vi "Launch Client.vi"(8 "error in":errorcluster, 10 "Client Name":string, 11 "Client Manager in":refnum<class "Client Manager.lvclass">) -> (0 "error out":errorcluster, 3 "Client Manager out":refnum<class "Client Manager.lvclass">)   [LabVIEW 2014, in "Client Manager.lvclass"]
uses:
  Client Manager.lvclass
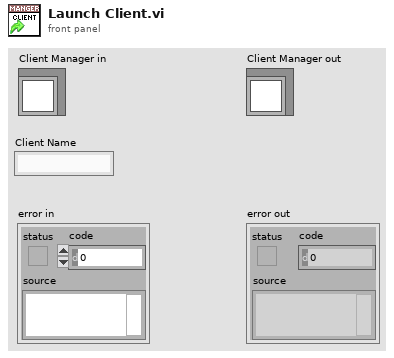
[diagram p1: front panel]
types:
  T1 = enum32{"Bad", "Idle", "Run top level", "Running"}
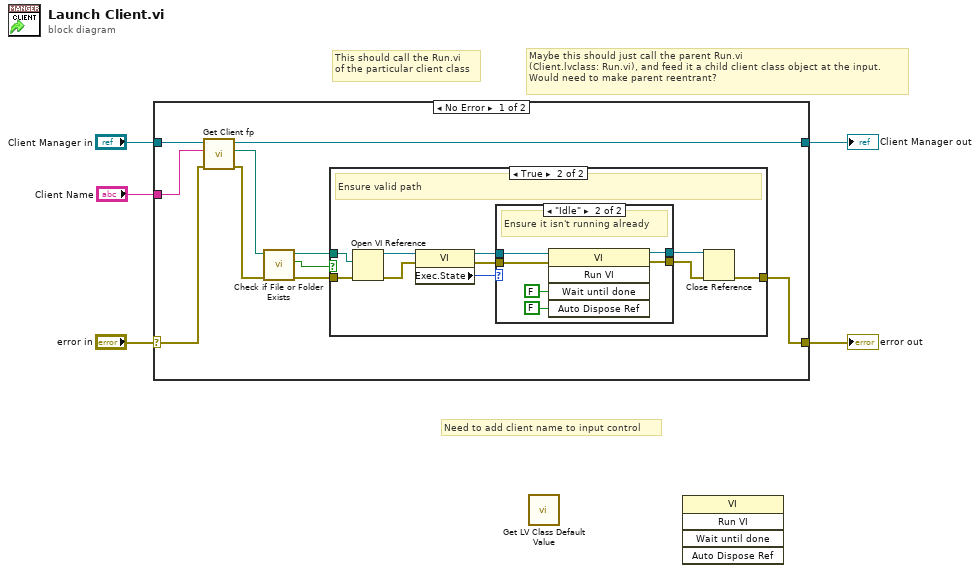
[diagram p0: block diagram]
diagram:
  # "Maybe this should just call the parent Run.vi \n(Client.lvclass: Run.vi), and feed it a child client class object at the input.\nWould need to make parent reentrant?"
  # "Need to add client name to input control"
  # "This should call the Run.vi\nof the particular client class"
  n1 = case shown="No Error" "error in" {
    selector: "error in" -> [w8 w36]
    tunnel: [w6 w36] -> w4
    tunnel: [w14 w35] -> w2
    tunnel: "Client Manager in" -> [w15 w35]
    tunnel: "Client Name" -> [w13 _]
    frame No Error {
      n2 = call "Get Client fp.vi"("error in"=w8, "Client Name"=w13, "Client Manager in"=w15) -> ("error out"=w7:errorcluster, "Client fp"=w12:path, "Client Manager out"=w14:refnum<class "Client Manager.lvclass">)  [unwired: 6 in]
      n3 = call <vilib>:"Check if File or Folder Exists.vi"("error in (no error)"=w7, "path"=w12) -> ("error out"=w9:errorcluster, "file or folder exists?"=w11:bool, "dup path"=w10:path)  [unwired: 7 in]
      n4 = case shown="True" w11 {
        tunnel: w10 -> [_ w26]
        tunnel: w9 -> [w16 w25]
        tunnel: [w16 w17] -> w6
        frame False {
        }
        frame True {
          # "Ensure valid path"
          n5 = Open VI Reference(vi path=w26, error in (no error)=w25) -> (vi reference=w24:refnum<vi>, error out=w23:errorcluster)  [unwired: 4 in]
          n6 = property class="VI"(reference=w24, error in=w23) -> (reference out=w21:refnum<vi>, error out=w20:errorcluster, "Exec.State"=w22:T1)
          n7 = case shown="\"Idle\"" w22 {
            tunnel: w21 -> [w28 w32]
            tunnel: w20 -> [w27 w31]
            tunnel: [w28 w30] -> w19
            tunnel: [w27 w29] -> w18
            frame Default {
            }
            frame "Idle" {
              # "Ensure it isn't running already"
              n8 = invoke class="VI" method="Run VI"(reference=w32, error in=w31, "Wait until done"=FALSE ("Wait Until Done"), "Auto Dispose Ref"=FALSE ("Auto Dispose Reference")) -> (reference out=w30:refnum<vi>, error out=w29:errorcluster)  [unwired: 1 in, 3 out]
            }
          }
          n9 = Close Reference(reference=w19, error in (no error)=w18) -> (error out=w17:errorcluster)
        }
      }
    }
    frame Error {
    }
  }
  "error out" <- w4
  "Client Manager out" <- w2
  n10 = call <vilib>:"Get LV Class Default Value.vi"() -> ()  [unwired: 10 in, 2 out]
  n11 = invoke class="VI" method="Run VI"() -> ()  [unwired: 5 in, 5 out]
